vi "标样核查配置.vi"() -> (2 "确认输出":bool, 3 "标样核查配置":T1={"数据保存间隔"=1.0, "水温标样值"=0.0, "pH标样值"=0.0, "溶解氧标样值"=0.0, "电导率标样值"=0.0, "浊度标样值"=0.0})   [LabVIEW 2016, in "国弘多参数.lvlib"]
uses:
  <vilib>/Utility/config.llb/NI_LVConfig.lvlib
panel:
  in  "浊度标样值":dbl caption="浊度"
  in  "电导率标样值":dbl caption="电导率"
  in  "溶解氧标样值":dbl caption="溶解氧"
  in  "pH标样值":dbl caption="pH"
  in  "水温标样值":dbl caption="水温"
  in  "取消":bool
  in  "确定":bool
  in  "数据保存间隔":dbl=1.0
  # "请输入数据保存间隔"
  # "min"
  # "请输入各参数标样值"
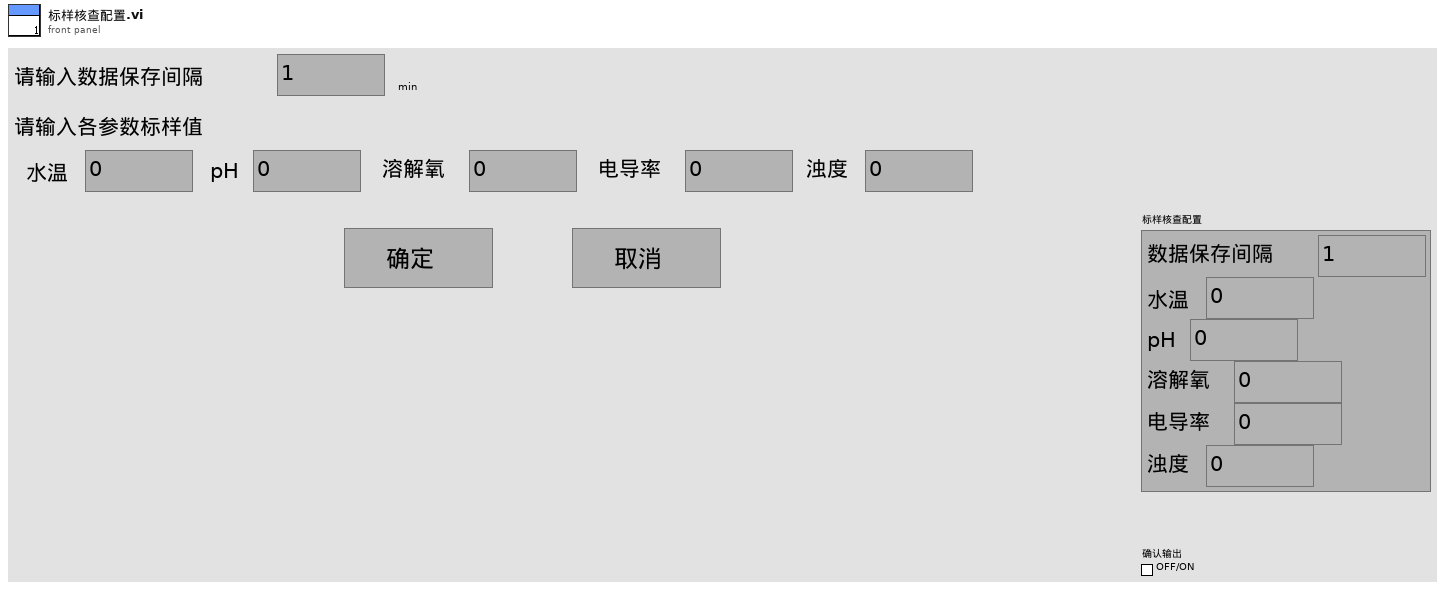
[diagram p1: front panel]
types:
  T1 = cluster{"数据保存间隔":dbl, "水温标样值":dbl, "pH标样值":dbl, "溶解氧标样值":dbl, "电导率标样值":dbl, "浊度标样值":dbl}
  T2 = typedef "NI_LVConfig.lvlib/Config Data RefNum.ctl" = refnum<k1>
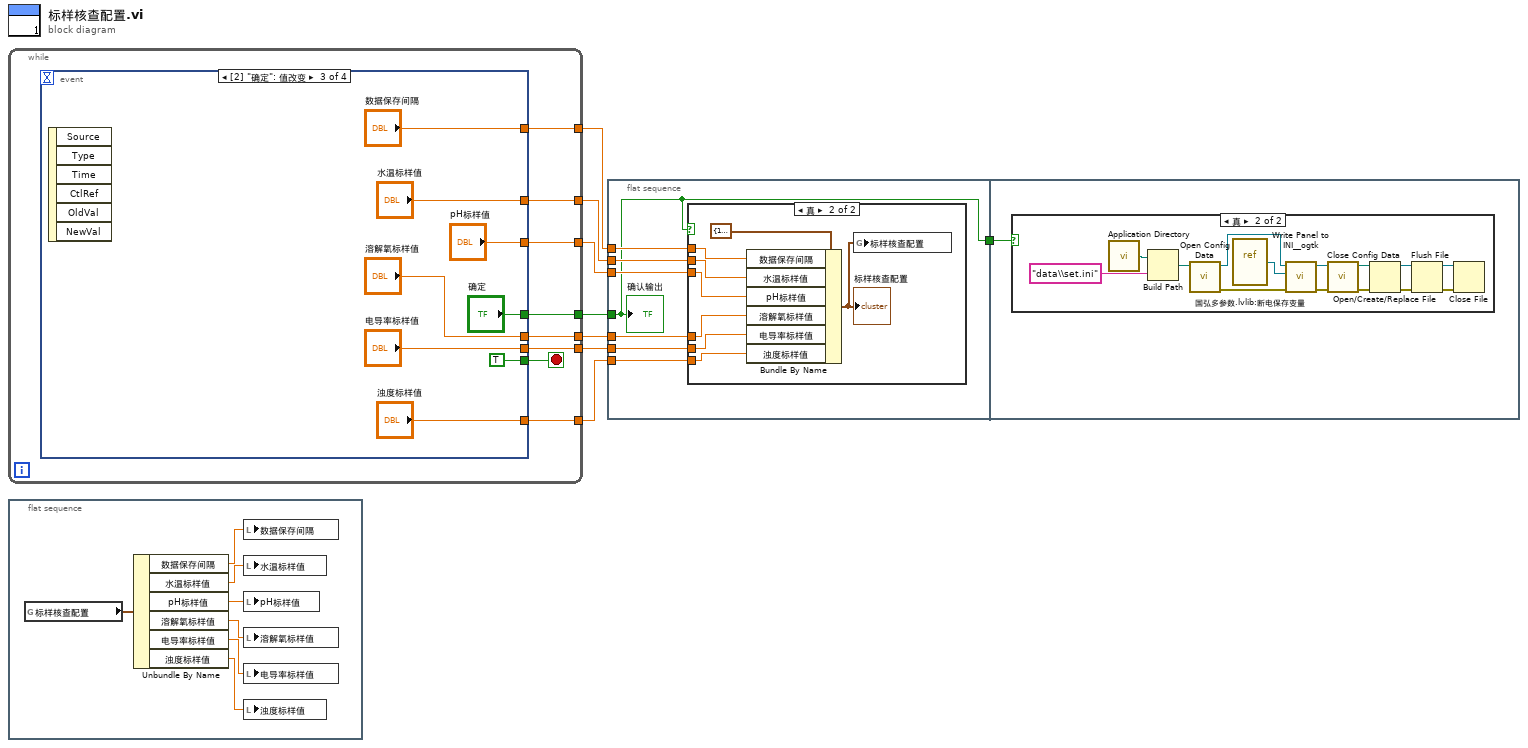
[diagram p0: block diagram]
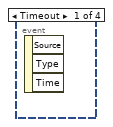
[diagram p4: hidden frame]
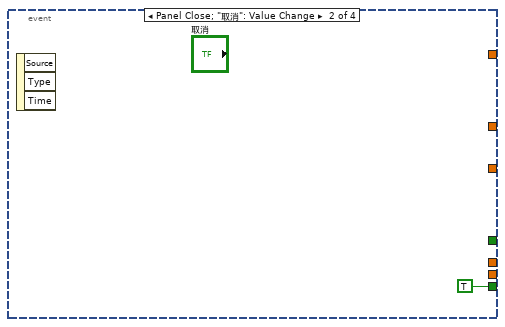
[diagram p5: hidden frame]
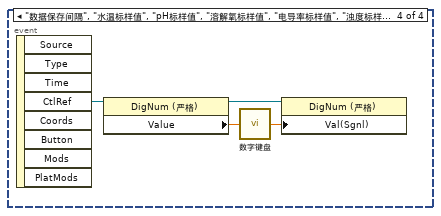
[diagram p6: hidden frame]
diagram:
  n1 = while {
    tunnel: [w15] -> w7
    tunnel: [w14] -> w8
    tunnel: [w13] -> w6
    tunnel: [w12] -> w5
    tunnel: [w11] -> w4
    tunnel: [w10] -> w3
    tunnel: [w9] -> w2
    stop <- w16 stop-if-true
    n2 = event shown="[2] \"确定\": 值改变" {
      selector: _ -> [_ _ _ _]
      dyn-events: _ -> [_ _ _ _]
      timeout: _ -> [_ _ _ _]
      tunnel: [_ TRUE TRUE _] -> w16
      tunnel: [_ _ "数据保存间隔" _] -> w15
      tunnel: [_ _ "确定" _] -> w14
      tunnel: [_ _ "水温标样值" _] -> w13
      tunnel: [_ _ "pH标样值" _] -> w12
      tunnel: [_ _ "溶解氧标样值" _] -> w11
      tunnel: [_ _ "电导率标样值" _] -> w10
      tunnel: [_ _ "浊度标样值" _] -> w9
      event Timeout {
        n3 = event-data() -> ()  [unwired: 1 in, 3 out]
      }
      event Panel Close; "取消": Value Change {
        n4 = event-data() -> ()  [unwired: 1 in, 3 out]
      }
      event "确定": Value Change {
        n5 = event-data() -> ()  [unwired: 1 in, 6 out]
      }
      event "数据保存间隔", "水温标样值", "pH标样值", "溶解氧标样值", "电导率标样值", "浊度标样值": Mouse Down {
        n6 = event-data() -> ("CtlRef"=w29:refnum<vi>)  [unwired: 1 in, 7 out]
        n7 = property class="DigNum (严格)"(reference=w29) -> (reference out=w26:refnum<vi>, "Value"=w28:dbl)  [unwired: 1 in, 1 out]
        n8 = call "数字键盘.vi"("OldNumber"=w28) -> ("NewNumber"=w27:sgl)
        n9 = property class="DigNum (严格)"(reference=w26, "Val(Sgnl)"=w27) -> ()  [unwired: 1 in, 2 out]
      }
    }
  }
  n10 = flat-sequence {
    frame #0 {
      n11 = global read "断电保存变量.vi" "标样核查配置"() -> (w36:T1)
      n12 = Unbundle By Name(w36) -> ("数据保存间隔"=w35:dbl, "水温标样值"=w30:dbl, "pH标样值"=w31:dbl, "溶解氧标样值"=w32:dbl, "电导率标样值"=w33:dbl, "浊度标样值"=w34:dbl)
      n13 = local write "数据保存间隔"(w35) -> ()
      n14 = local write "水温标样值"(w30) -> ()
      n15 = local write "pH标样值"(w31) -> ()
      n16 = local write "溶解氧标样值"(w32) -> ()
      n17 = local write "电导率标样值"(w33) -> ()
      n18 = local write "浊度标样值"(w34) -> ()
    }
  }
  n19 = flat-sequence {
    tunnel: w8 -> [w37]
    tunnel: w7 -> [w43]
    tunnel: w6 -> [w42]
    tunnel: w5 -> [w41]
    tunnel: w4 -> [w40]
    tunnel: w3 -> [w39]
    tunnel: w2 -> [w38]
    tunnel: [w37] -> w1
    tunnel: w1 -> [w52]
    frame #0 {
      n20 = case shown="真" w37 {
        tunnel: w43 -> [_ w50]
        tunnel: w42 -> [_ w49]
        tunnel: w41 -> [_ w48]
        tunnel: w40 -> [_ w47]
        tunnel: w39 -> [_ w46]
        tunnel: w38 -> [_ w45]
        frame False {
        }
        frame True {
          n21 = Bundle By Name(cluster=T1 {"数据保存间隔"=1.0, "水温标样值"=0.0, "pH标样值"=0.0, "溶解氧标样值"=0.0, "电导率标样值"=0.0, "浊度标样值"=0.0} ("标样核查配置"), "数据保存间隔"=w50, "水温标样值"=w49, "pH标样值"=w48, "溶解氧标样值"=w47, "电导率标样值"=w46, "浊度标样值"=w45) -> (w44:T1)
          "标样核查配置" <- w44
          n22 = global write "断电保存变量.vi" "标样核查配置"(w44) -> ()
        }
      }
      "确认输出" <- w37
    }
    frame #1 {
      n23 = case shown="真" w52 {
        frame False {
        }
        frame True {
          n24 = call <vilib>:"Application Directory.vi"() -> ("Application Directory"=w57:path)
          n25 = Build Path(base path=w57, name or relative path="data\\set.ini" ("名称或相对路径")) -> (appended path=w58:path)
          n26 = call <vilib>:"Open Config Data.vi"("configuration file path"=w58) -> ("error out"=w54:errorcluster, "refnum"=w53:T2)  [unwired: 8 in, 1 out]
          n27 = vi-ref "国弘多参数.lvlib:断电保存变量.vi"() -> (w60:refnum<vi>)
          n28 = call <userlib>:"Write Panel to INI__ogtk.vi"("error in (no error)"=w54, "VI ref"=w60, "refnum"=w53) -> ("error out"=w56:errorcluster, "refnum out"=w55:T2)  [unwired: 7 in]
          n29 = call <vilib>:"Close Config Data.vi"("error in (no error)"=w56, "refnum"=w55) -> ("error out"=w64:errorcluster, "file path"=w63:path)  [unwired: 8 in]
          n30 = Open/Create/Replace File(file path (use dialog)=w63, error in=w64) -> (refnum out=w62:refnum<file>, error out=w61:errorcluster)  [unwired: 4 in, 1 out]
          n31 = Flush File(refnum=w62, error in=w61) -> (refnum out=w66:refnum<file>, error out=w65:errorcluster)
          n32 = Close File(refnum=w66, error in=w65) -> ()  [unwired: 2 out]
        }
      }
    }
  }
